vi "Permute.vi"(1 "k":u32, 2 "n":u32) -> (0 "nPk":dbl)   [LabVIEW 2020, in "NI_Gmath.lvlib"]
doc: "Computes the number of ways to obtain an ordered subset of <B>k</B> elements from a set of <B>n</B> elements."
uses:
  NI_Gmath.lvlib
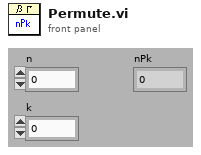
[diagram p1: front panel]
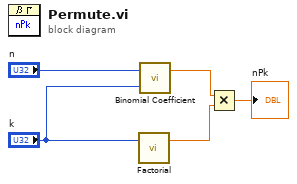
[diagram p0: block diagram]
diagram:
  n1 = call "Factorial.vi"("n"="k") -> ("n!"=w4:dbl)  [unwired: 2 in]
  n2 = call "Binomial Coefficient.vi"("k"="k", "n"="n") -> ("binomial coefficient (n,k)"=w5:dbl)  [unwired: 1 out]
  n3 = Multiply(x=w5, y=w4) -> (x*y=→"nPk":dbl)
